vi "DC_CUR_VOLT_test.vi"() -> ()   [LabVIEW 2018]
uses:
  <instrlib>/niDCPower/nidcpower.llb/niDCPower Source Mode.ctl
  <instrlib>/niDCPower/nidcpower.llb/niDCPower Output Function.ctl
panel:
  out "curmes_V_MB, A 2":dbl=1.286582923181595e-06
  out "voltmes_V_MB, V 2":dbl=-0.0008111687136758278 caption="measurement" format="%_6g"
  out "chart_1 3":dbl(graph)=-0.0008111687136758278 caption="Waveform Chart 5"
  in  "V_MB, V 2":dbl=-1.0 caption="voltage level" format="%_6p"
  in  "curlim_V_MB, A 2":dbl=0.009999999999999998 caption="current limit" min=0.0 format="%_6p"
  in  "current level range":dbl=0.001 format="%#.6p"
  out "curmes_V_MB, A":dbl=4.935234870429662e-05
  out "voltmes_V_MB, V":dbl=-0.00022454272865531083 caption="measurement" format="%_6g"
  out "chart_1 2":dbl(graph)=-0.00022454272865531083 caption="Waveform Chart 5"
  in  "V_MB, V":dbl=6.0 caption="voltage level" format="%_6p"
  in  "curlim_V_MB, A":dbl=0.3 caption="current limit" min=0.0 format="%_6p"
  out "curmes_I_LED, A":dbl=-1.0475074862280678e-06
  in  "Resource Name":refnum<k15>="PXI1Slot3" caption="Источник питания"
  out "Power off":bool=TRUE
  in  "POWER":bool
  in  "voltlim_I_LED, V":dbl=10.0 caption="current limit" min=0.01 format="%_6p"
  in  "I_LED, A":dbl=0.005 caption="voltage level" format="%_6p"
  out "chart_1":dbl(graph)=-1.0475074862280678e-06 caption="Waveform Chart 5"
  out "voltmes_I_LED, V":dbl=0.00036230164453815835 caption="measurement" format="%_6g"
  in  "Стоп":bool
  # "ch0"
  # "ch1"
  # "ch2"
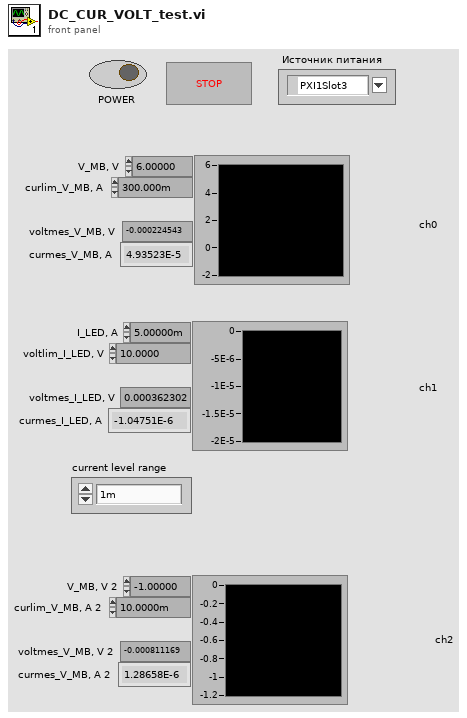
[diagram p1: front panel]
types:
  T1 = typedef "niDCPower Output Function.ctl" = i32
  T2 = typedef "niDCPower Source Mode.ctl" = i32
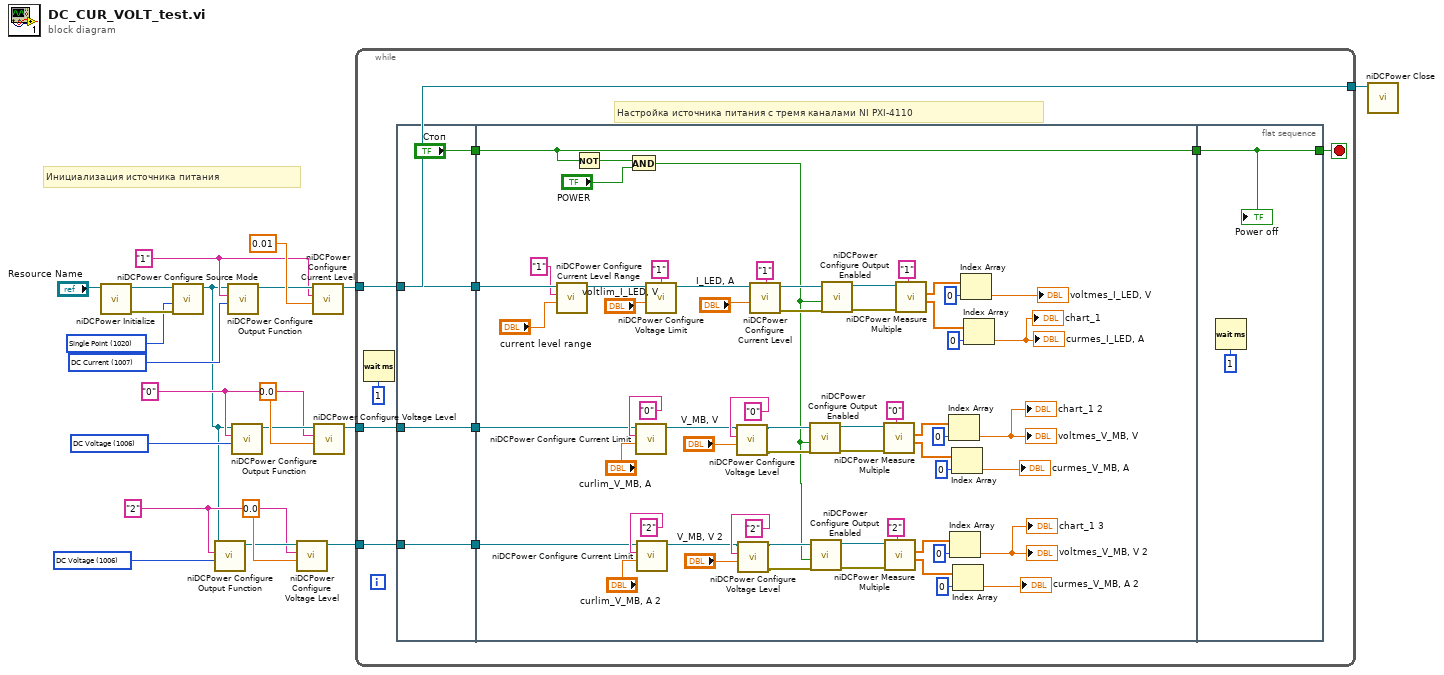
[diagram p0: block diagram]
diagram:
  w4 = T1 1006 items=["DC Voltage"=1006, "DC Current"=1007, "Pulse Voltage"=1049, "Pulse Current"=1050] ("output function")
  w3 = "2"
  w9 = T1 1006 items=["DC Voltage"=1006, "DC Current"=1007, "Pulse Voltage"=1049, "Pulse Current"=1050] ("output function")
  w8 = "0"
  w12 = T1 1007 items=["DC Voltage"=1006, "DC Current"=1007, "Pulse Voltage"=1049, "Pulse Current"=1050] ("output function")
  w17 = T2 1020 items=["Single Point"=1020, "Sequence"=1021] ("source mode")
  w13 = "1"
  # "Инициализация источника питания"
  n1 = call <instrlib>:"niDCPower Initialize.vi"("resource name"="Resource Name") -> ("error out"=w18:errorcluster, "instrument handle out"=w19:refnum<k15>)  [unwired: 3 in, 6 out]
  n2 = call <instrlib>:"niDCPower Configure Source Mode.vi"("error in (no error)"=w18, "source mode"=w17, "instrument handle"=w19) -> ("instrument handle out"=w1:refnum<k15>)  [unwired: 8 out]
  n3 = call <instrlib>:"niDCPower Configure Output Function.vi"("output function"=w4, "channel name"=w3, "instrument handle"=w1) -> ("instrument handle out"=w5:refnum<k15>)  [unwired: 7 in, 1 out]
  n4 = call <instrlib>:"niDCPower Configure Output Function.vi"("output function"=w12, "channel name"=w13, "instrument handle"=w1) -> ("instrument handle out"=w14:refnum<k15>)  [unwired: 7 in, 1 out]
  n5 = call <instrlib>:"niDCPower Configure Output Function.vi"("output function"=w9, "channel name"=w8, "instrument handle"=w1) -> ("instrument handle out"=w10:refnum<k15>)  [unwired: 7 in, 1 out]
  n6 = call <instrlib>:"niDCPower Configure Voltage Level.vi"("voltage level"=0.0, "channel name"=w3, "instrument handle"=w5) -> ("instrument handle out"=w2:refnum<k15>)  [unwired: 7 in, 1 out]
  n7 = call <instrlib>:"niDCPower Configure Current Level.vi"("current level"=0.01, "channel name"=w13, "instrument handle"=w14) -> ("instrument handle out"=w16:refnum<k15>)  [unwired: 7 in, 1 out]
  n8 = call <instrlib>:"niDCPower Configure Voltage Level.vi"("voltage level"=0.0, "channel name"=w8, "instrument handle"=w10) -> ("instrument handle out"=w7:refnum<k15>)  [unwired: 7 in, 1 out]
  n9 = while {
    tunnel: w16 -> [w26]
    tunnel: [w26] -> w15
    tunnel: w7 -> [w24]
    tunnel: w2 -> [w22]
    stop <- w27 stop-if-true
    # "Настройка источника питания с тремя каналами NI PXI-4110"
    n10 = Wait (ms)(milliseconds to wait=u32 1) -> ()  [unwired: 1 out]
    n11 = flat-sequence {
      tunnel: ["Стоп"] -> w30
      tunnel: [w34] -> w28
      tunnel: w26 -> [w34]
      tunnel: [w33] -> w25
      tunnel: w24 -> [w33]
      tunnel: [w32] -> w23
      tunnel: w22 -> [w32]
      tunnel: w30 -> [w93]
      tunnel: [w93] -> w29
      tunnel: w28 -> [w58]
      tunnel: w25 -> [w54]
      tunnel: w23 -> [w36]
      tunnel: [w95] -> w27
      tunnel: w29 -> [w95]
      frame #0 {
      }
      frame #1 {
        n12 = call <instrlib>:"niDCPower Configure Current Level Range.vi"("current level range"="current level range", "channel name"="1", "instrument handle"=w58) -> ("instrument handle out"=w57:refnum<k15>)  [unwired: 7 in, 1 out]
        n13 = Not(x=w93) -> (.not. x?=w92:bool)
        n14 = And(x=w92, y="POWER") -> (x .and. y?=w37:bool)
        n15 = call <instrlib>:"niDCPower Configure Current Limit.vi"("current limit"="curlim_V_MB, A", "channel name"="0", "instrument handle"=w54) -> ("instrument handle out"=w61:refnum<k15>)  [unwired: 7 in, 1 out]
        n16 = call <instrlib>:"niDCPower Configure Current Limit.vi"("current limit"="curlim_V_MB, A 2", "channel name"="2", "instrument handle"=w36) -> ("instrument handle out"=w40:refnum<k15>)  [unwired: 7 in, 1 out]
        n17 = call <instrlib>:"niDCPower Configure Voltage Limit.vi"("voltage limit"="voltlim_I_LED, V", "channel name"="1", "instrument handle"=w57) -> ("instrument handle out"=w87:refnum<k15>)  [unwired: 7 in, 1 out]
        n18 = call <instrlib>:"niDCPower Configure Voltage Level.vi"("voltage level"="V_MB, V", "channel name"="0", "instrument handle"=w61) -> ("error out"=w66:errorcluster, "instrument handle out"=w65:refnum<k15>)  [unwired: 7 in]
        n19 = call <instrlib>:"niDCPower Configure Voltage Level.vi"("voltage level"="V_MB, V 2", "channel name"="2", "instrument handle"=w40) -> ("error out"=w44:errorcluster, "instrument handle out"=w43:refnum<k15>)  [unwired: 7 in]
        n20 = call <instrlib>:"niDCPower Configure Current Level.vi"("current level"="I_LED, A", "channel name"="1", "instrument handle"=w87) -> ("error out"=w85:errorcluster, "instrument handle out"=w88:refnum<k15>)  [unwired: 7 in]
        n21 = call <instrlib>:"niDCPower Configure Output Enabled.vi"("error in (no error)"=w66, "output enabled"=w37, "instrument handle"=w65) -> ("error out"=w74:errorcluster, "instrument handle out"=w75:refnum<k15>)  [unwired: 7 in]
        n22 = call <instrlib>:"niDCPower Configure Output Enabled.vi"("error in (no error)"=w44, "output enabled"=w37, "instrument handle"=w43) -> ("error out"=w52:errorcluster, "instrument handle out"=w53:refnum<k15>)  [unwired: 7 in]
        n23 = call <instrlib>:"niDCPower Configure Output Enabled.vi"("error in (no error)"=w85, "output enabled"=w37, "instrument handle"=w88) -> ("error out"=w82:errorcluster, "instrument handle out"=w83:refnum<k15>)  [unwired: 7 in]
        n24 = call <instrlib>:"niDCPower Measure Multiple.vi"("error in (no error)"=w74, "channel name"="0", "instrument handle"=w75) -> ("current measurements"=w69:dbl[], "voltage measurements"=w72:dbl[])  [unwired: 5 in, 2 out]
        n25 = call <instrlib>:"niDCPower Measure Multiple.vi"("error in (no error)"=w52, "channel name"="2", "instrument handle"=w53) -> ("current measurements"=w47:dbl[], "voltage measurements"=w50:dbl[])  [unwired: 5 in, 2 out]
        n26 = call <instrlib>:"niDCPower Measure Multiple.vi"("error in (no error)"=w82, "channel name"="1", "instrument handle"=w83) -> ("current measurements"=w77:dbl[], "voltage measurements"=w80:dbl[])  [unwired: 5 in, 2 out]
        n27 = Index Array(array=w72, index=0) -> (element=→"chart_1 2" →"voltmes_V_MB, V":dbl)
        n28 = Index Array(array=w50, index=0) -> (element=→"chart_1 3" →"voltmes_V_MB, V 2":dbl)
        n29 = Index Array(array=w69, index=0) -> (element=→"curmes_V_MB, A":dbl)
        n30 = Index Array(array=w47, index=0) -> (element=→"curmes_V_MB, A 2":dbl)
        n31 = Index Array(array=w80, index=0) -> (element=→"voltmes_I_LED, V":dbl)
        n32 = Index Array(array=w77, index=0) -> (element=→"chart_1" →"curmes_I_LED, A":dbl)
      }
      frame #2 {
        n33 = Wait (ms)(milliseconds to wait=u32 1) -> ()  [unwired: 1 out]
        "Power off" <- w95
      }
    }
  }
  n34 = call <instrlib>:"niDCPower Close.vi"("instrument handle"=w15) -> ()  [unwired: 10 in, 1 out]
